vi "Theta 1.vi"(5 "XYZ_60":dbl[](array[numeric])=[0.0, 0.0, 0.0], 7 "XYZ_0":dbl[](array[numeric])=[0.0, 0.0, 0.0], 9 "theta_2":dbl, 10 "theta_0":dbl, 11 "6R Type 2 Serial Arm Class in":refnum<class "NI_Robotics_6R Type 2 Serial Arm Class.lvclass">) -> (1 "Valid":bool, 2 "theta1":dbl, 3 "6R Type 2 Serial Arm Class out":refnum<class "NI_Robotics_6R Type 2 Serial Arm Class.lvclass">)   [LabVIEW 2017, in "NI_Robotics_6R Type 2 Serial Arm Class.lvclass"]
uses:
  <vilib>/robotics/Kinematics/Analytical/6R/Type 2/NI_Robotics_6R Type 2 Serial Arm Class.lvclass
  c:/Program Files (x86)/National Instruments/LabVIEW 2017/vi.lib/robotics/Kinematics/Analytical/Generic/NI_Robotics_Analytical Serial Arm Class.lvclass
  <vilib>/robotics/Kinematics/Link/NI_Robotics_Link.lvclass/NI_Robotics_Link.ctl
  <vilib>/Analysis/7linalg.llb/Solve Linear Equations (single right hand).vi
  <vilib>/robotics/Kinematics/Link/Get Kinematic Parameters.vi
  <vilib>/Analysis/baseanly.llb/Solve Linear Equations By Cholesky.vi
  <vilib>/Analysis/baseanly.llb/Real Matrix to Compact Array.vi
  <vilib>/Analysis/baseanly.llb/Real Compact Tri-Matrix Linear Eqs.vi
  <vilib>/robotics/Kinematics/Analytical/Generic/NI_Robotics_Analytical Serial Arm Class.lvclass
  c:/Program Files (x86)/National Instruments/LabVIEW 2017/vi.lib/robotics/Kinematics/Robot/NI_Robotics_Serial Robot Arm.lvclass
  <vilib>/Analysis/7linalg.llb/Solve Linear Eqs (General).vi
  <vilib>/Analysis/7linalg.llb/Solve Linear Eqs (Gen, single right hand).vi
  <vilib>/robotics/Kinematics/Analytical/Generic/Accessors/Read alpha_n0.vi
  <vilib>/robotics/Kinematics/Robot/Get Links.vi
  <vilib>/Analysis/NI_AALPro.lvlib
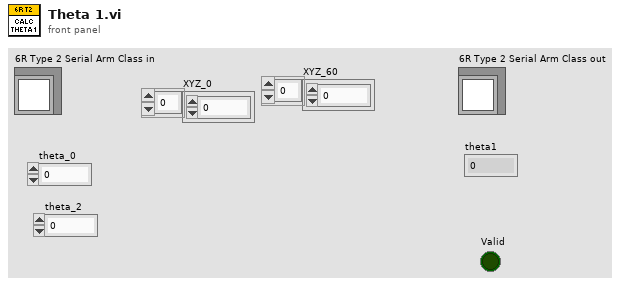
[diagram p1: front panel]
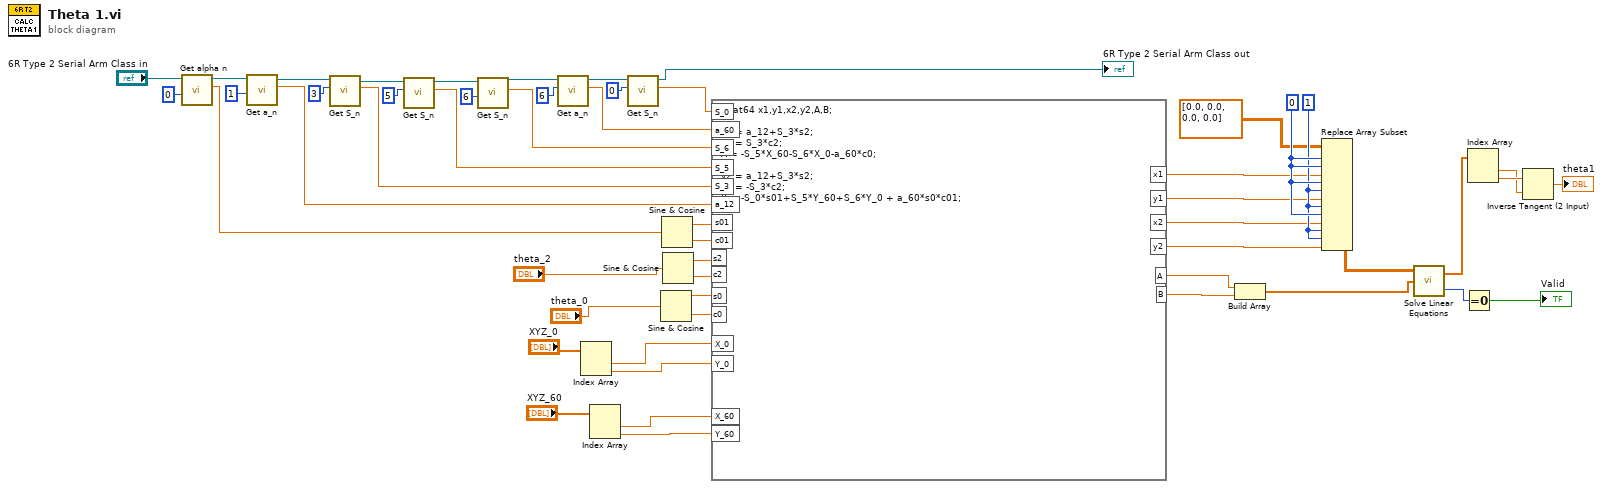
[diagram p0: block diagram]
diagram:
  w17 = 1 ("disabled index (col)")
  w18 = 0 ("index (row)")
  n1 = call <vilib>:"Get alpha n.vi"("n"=0, "Analytical Serial Arm Class in"="6R Type 2 Serial Arm Class in") -> ("alpha n"=w19:dbl, "Analytical Serial Arm Class out"=w23:refnum<class "NI_Robotics_6R Type 2 Serial Arm Class.lvclass">)  [unwired: 8 in]
  n2 = call <vilib>:"Get a_n.vi"("n"=1, "Analytical Serial Arm Class in"=w23) -> ("a_n"=w31:dbl, "Analytical Serial Arm Class out"=w52:refnum<class "NI_Robotics_6R Type 2 Serial Arm Class.lvclass">)  [unwired: 8 in]
  n3 = call <vilib>:"Get S_n.vi"("n"=3, "Analytical Serial Arm Class in"=w52) -> ("S_n"=w32:dbl, "Analytical Serial Arm Class out"=w50:refnum<class "NI_Robotics_6R Type 2 Serial Arm Class.lvclass">)  [unwired: 8 in]
  n4 = call <vilib>:"Get S_n.vi"("n"=5, "Analytical Serial Arm Class in"=w50) -> ("S_n"=w33:dbl, "Analytical Serial Arm Class out"=w48:refnum<class "NI_Robotics_6R Type 2 Serial Arm Class.lvclass">)  [unwired: 8 in]
  n5 = call <vilib>:"Get S_n.vi"("n"=6, "Analytical Serial Arm Class in"=w48) -> ("S_n"=w34:dbl, "Analytical Serial Arm Class out"=w46:refnum<class "NI_Robotics_6R Type 2 Serial Arm Class.lvclass">)  [unwired: 8 in]
  n6 = call <vilib>:"Get a_n.vi"("n"=6, "Analytical Serial Arm Class in"=w46) -> ("a_n"=w35:dbl, "Analytical Serial Arm Class out"=w44:refnum<class "NI_Robotics_6R Type 2 Serial Arm Class.lvclass">)  [unwired: 8 in]
  n7 = Index Array(array="XYZ_0") -> (element #1=w29:dbl, element #2=w28:dbl)  [unwired: 2 in]
  n8 = Index Array(array="XYZ_60") -> (element #1=w26:dbl, element #2=w25:dbl)  [unwired: 2 in]
  n9 = call <vilib>:"Get S_n.vi"("n"=0, "Analytical Serial Arm Class in"=w44) -> ("S_n"=w42:dbl, "Analytical Serial Arm Class out"=→"6R Type 2 Serial Arm Class out":refnum<class "NI_Robotics_6R Type 2 Serial Arm Class.lvclass">)  [unwired: 8 in]
  n10 = Sine & Cosine(0:"theta_0") -> (1:w37:dbl, 2:w38:dbl)
  n11 = Sine & Cosine(0:w19) -> (1:w21:dbl, 2:w20:dbl)
  n12 = Sine & Cosine(0:"theta_2") -> (1:w40:dbl, 2:w41:dbl)
  n13 = formula code="float64 x1,y1,x2,y2,A,B;\n\nx1 = a_12+S_3*s2;\ny1 = S_3*c2;\nA = -S_5*X_60-S_6*X_0-a_60*c0;\n\ny2 = a_12+S_3*s2;\nx2 = -S_3*c2;\nB = -S_0*s01+S_5*Y_60+S_6*Y_0 + a_60*s0*c01;"("S_0"=w42, "a_60"=w35, "S_6"=w34, "S_5"=w33, "S_3"=w32, "a_12"=w31, "s2"=w40, "c2"=w41, "s0"=w37, "c0"=w38, "X_0"=w29, "Y_0"=w28, "X_60"=w26, "Y_60"=w25, "s01"=w21, "c01"=w20) -> ("x1"=w15:dbl, "y1"=w12:dbl, "x2"=w13:dbl, "y2"=w14:dbl, "A"=w11:dbl, "B"=w10:dbl)
  n14 = Build Array(w11, w10) -> (w8:dbl[])
  n15 = Replace Array Subset(array=dbl[][] [[0.0, 0.0], [0.0, 0.0]], new element #1=w15, index (row) #1=w18, index (col) #1=w18, new element #2=w12, index (row) #2=w18, index (col) #2=w17, new element #3=w13, index (row) #3=w17, index (col) #3=w18, new element #4=w14, index (row) #4=w17, index (col) #4=w17) -> (w9:dbl[][])
  n16 = call-poly <vilib>:"Solve Linear Equations.vi"("Known Vector"=w8, "Input Matrix"=w9) -> ("error"=w7:i32, "Solution Vector"=w3:dbl[])  [unwired: 1 in]
  n17 = Equal To 0?(x=w7) -> (x = 0?=→"Valid":bool)
  n18 = Index Array(array=w3) -> (element #1=w4:dbl, element #2=w5:dbl)  [unwired: 2 in]
  n19 = Inverse Tangent (2 Input)(1:w4, 2:w5) -> (0:→"theta1":dbl)
